vi "Test Bitwise OR.vi"(8 "error in (no error)":errorcluster, 11 "Test Case In":refnum<class "01_Image.lvclass">) -> (0 "error out":errorcluster, 3 "Test Case Out":refnum<class "01_Image.lvclass">)   [LabVIEW 2020, in "test.lvlib" / "01_Image.lvclass"]
uses:
  01_Image.lvclass
  C:/Program Files (x86)/National Instruments/LabVIEW 2026/vi.lib/Astemes/LUnit/Test Case.lvclass
  common/Image Size (Integer).ctl
  image/In-Range Image Grey Range.ctl
  <vilib>/Astemes/LUnit/Test Case.lvclass/Test Case.ctl
  image/New Image (Greyscale Preallocated).vi
  4993e8ee-a06a-463a-9684-69129f64d5ce.vi
  image/New Image (Greyscale Preallocated).vi/6598b9e0-8a08-46f5-91fd-ca1b87217137.vi
  image/Match-Value Image (Greyscale).vi/0720c4fc-c714-46e4-a6a5-fc7e731e80c2.vi
  image/In-Range (Greyscale).vi/5701baee-35e2-4306-9a77-a9fdbb5b3a7f.vi
  image/Bitwise OR (Greyscale with Mask).vi/0e84d7da-7af3-4d73-801a-9d94e7981347.vi
  image/Draw Image to Picture (Greyscale).vi/9ae995ca-ccda-485c-89ac-02736fde3e8e.vi
  <vilib>/Astemes/LUnit/Core/LUnit Test Case/Private/Append Pass Result.vi
  <vilib>/Astemes/LUnit/Core/LUnit Test Case/Private/Append Fail Result.vi
  4993e8ee-a06a-463a-9684-69129f64d5ce.vi/9c5d11cd-9439-4240-a1ee-d9baace9c924.vi
  <vilib>/Astemes/LUnit/Core/LUnit Test Case/Private/Run In UI.vi
  <vilib>/Utility/error.llb/Clear Errors.vi
  <vilib>/Utility/error.llb/Error Cluster From Error Code.vi
  image/image.lvlib
  common/common.lvlib
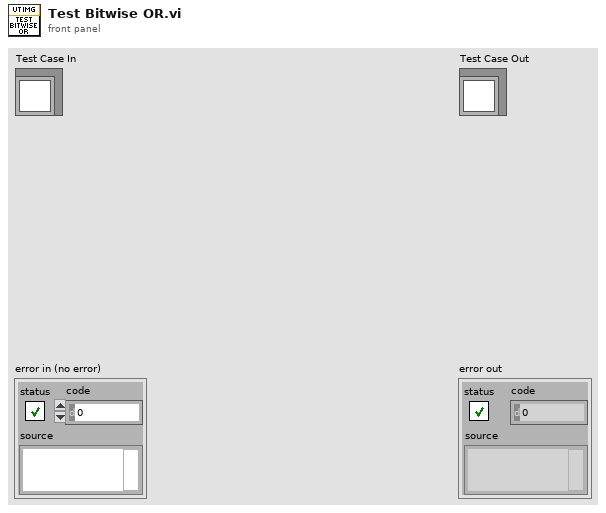
[diagram p1: front panel]
types:
  T1 = typedef "image.lvlib/In-Range Image Grey Range.ctl" = cluster{"Lower":u8, "Upper":u8}
  T2 = typedef "common.lvlib/Image Size (Integer).ctl" = cluster{"Width":u16, "Height":u16}
  T3 = typedef "image.lvlib/Greyscale Image.ctl" = refnum<data-value>
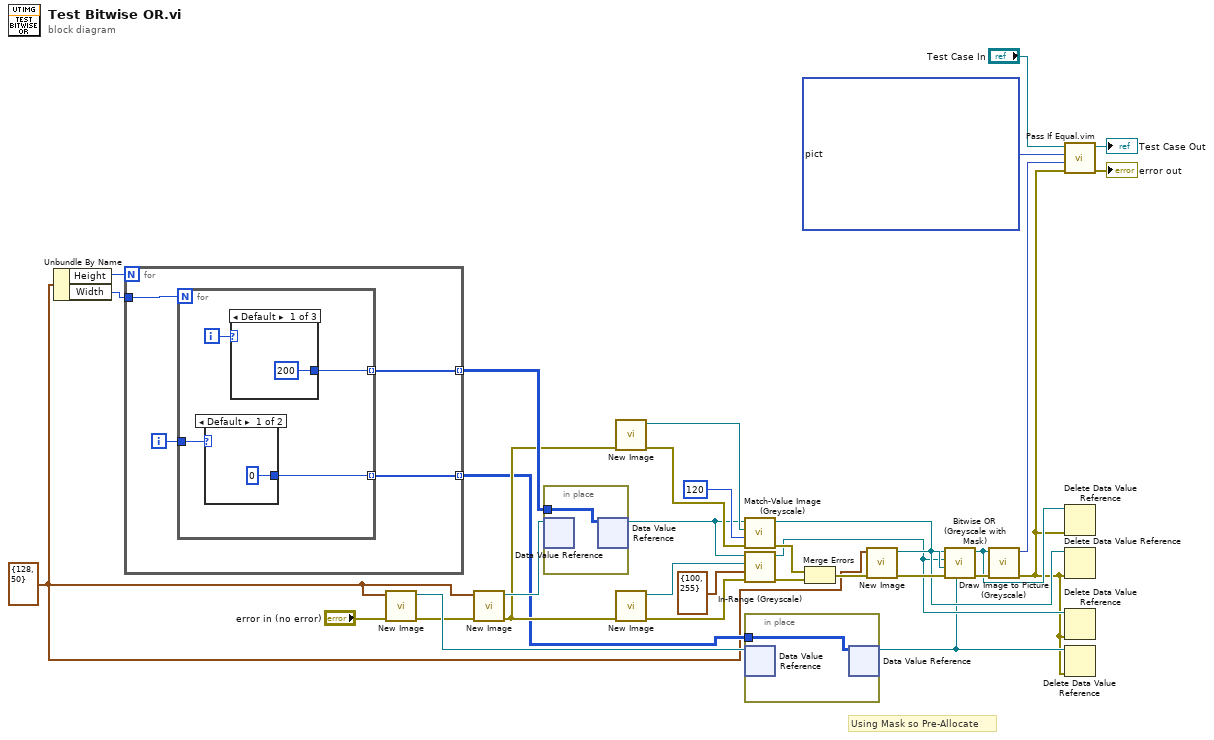
[diagram p0: block diagram]
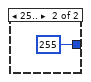
[diagram p2: hidden frame]
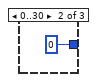
[diagram p3: hidden frame]
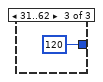
[diagram p4: hidden frame]
diagram:
  w1 = T2 {"Width"=128, "Height"=50} ("Preallocated Image Size (Default 0,0)")
  # "Using Mask so Pre-Allocate"
  n1 = Unbundle By Name(w1) -> ("Height"=w30:u16, "Width"=w29:u16)
  n2 = for {
    N: w30 -> [_]
    tunnel: [w37] -> w27 mode=indexing
    tunnel: w29 -> [w36]
    tunnel: [w35] -> w18 mode=indexing
    i -> [w34]
    n3 = for {
      N: w36 -> [_]
      tunnel: [w40] -> w37 mode=indexing
      tunnel: [w39] -> w35 mode=indexing
      tunnel: w34 -> [w38]
      i -> [w41]
      n4 = case shown="Default" w38 {
        tunnel: [u8 0 u8 255] -> w39
        frame Default {
        }
        frame 25.. {
        }
      }
      n5 = case shown="Default" w41 {
        tunnel: [u8 200 u8 0 u8 120] -> w40
        frame Default {
        }
        frame 0..30 {
        }
        frame 31..62 {
        }
      }
    }
  }
  n6 = call-poly "New Image.vi"("error in (no error)"="error in (no error)", "Preallocated Image Size (Default 0,0)"=w1) -> ("error out"=w10:errorcluster, "Greyscale Image"=w19:T3)  [unwired: 8 in]
  n7 = call-poly "New Image.vi"("error in (no error)"=w10, "Preallocated Image Size (Default 0,0)"=w1) -> ("error out"=w24:errorcluster, "Greyscale Image"=w28:T3)  [unwired: 8 in]
  n8 = in-place {
    in-place-border: w27 -> [w47]
    n9 = in-place-dvr #1(w28) -> ()  [unwired: 2 out]
    n10 = in-place-dvr #1(w47) -> (w16:T3)  [unwired: 1 out]
  }
  n11 = call-poly "New Image.vi"("error in (no error)"=w24) -> ("error out"=w25:errorcluster, "Greyscale Image"=w17:T3)  [unwired: 9 in]
  n12 = call-poly "New Image.vi"("error in (no error)"=w24) -> ("error out"=w14:errorcluster, "Greyscale Image"=w15:T3)  [unwired: 9 in]
  n13 = call "Match-Value Image (Greyscale).vi"("error in (no error)"=w25, "Value"=u8 120, "Match in"=w17, "Greyscale Image-Source in"=w16) -> ("error out"=w23:errorcluster, "Match in"=w5:T3)  [unwired: 6 in]
  n14 = call "In-Range (Greyscale).vi"("error in (no error)"=w14, "In-Range Image Colour Range"=T1 {"Lower"=100, "Upper"=255}, "In-Range-Result in"=w15, "Greyscale Image-Source in"=w16) -> ("error out"=w13:errorcluster, "In-Range-Result"=w4:T3)  [unwired: 6 in]
  n15 = in-place {
    in-place-border: w18 -> [w48]
    n16 = in-place-dvr #2(w19) -> ()  [unwired: 2 out]
    n17 = in-place-dvr #2(w48) -> (w3:T3)  [unwired: 1 out]
  }
  n18 = Merge Errors(w23, w13) -> (w22:errorcluster)
  n19 = call-poly "New Image.vi"("error in (no error)"=w22, "Preallocated Image Size (Default 0,0)"=w1) -> ("error out"=w21:errorcluster, "Greyscale Image"=w20:T3)  [unwired: 8 in]
  n20 = call "Bitwise OR (Greyscale with Mask).vi"("Mask in"=w3, "error in (no error)"=w21, "Greyscale Image Destination in"=w20, "Greyscale Image B in"=w4, "Greyscale Image A in"=w5) -> ("error out"=w11:errorcluster, "Greyscale Image Destination"=w6:T3)  [unwired: 5 in]
  n21 = call "Draw Image to Picture (Greyscale).vi"("error in (no error)"=w11, "Greyscale Image Source in"=w6) -> ("error out"=w2:errorcluster, "Picture"=w9:picture)  [unwired: 8 in]
  n22 = call "Pass If Equal.vim"("error in (no error)"=w2, "Actual"=w9, "Expected"=picture bytes[8480] ("Picture"), "LUnit Test Case In"="Test Case In") -> ("error out"=→"error out":errorcluster, "LUnit Test Case Out"=→"Test Case Out":refnum<class "01_Image.lvclass">)  [unwired: 6 in]
  n23 = Delete Data Value Reference(data value reference=w6, error in=w2) -> ()  [unwired: 2 out]
  n24 = Delete Data Value Reference(data value reference=w5, error in=w2) -> ()  [unwired: 2 out]
  n25 = Delete Data Value Reference(data value reference=w4, error in=w2) -> ()  [unwired: 2 out]
  n26 = Delete Data Value Reference(data value reference=w3, error in=w2) -> ()  [unwired: 2 out]
